vi "calcRigidBodyAuth.vi"(8 "error in (no error)":errorcluster, 10 "Rigid Body Stroke File":string="rbStroke.txt", 11 "OptCtrl in":refnum<class "OptCtrl.lvclass">) -> (0 "error out":errorcluster, 2 "Authority (1 um)":dbl[](array[numeric]), 3 "OptCtrl out":refnum<class "OptCtrl.lvclass">)   [LabVIEW 2016, in "OfcFunc.lvlib" / "OptCtrl.lvclass"]
doc: "Calculate the distribution of control authority of rigid body."
uses:
  OptCtrl.lvclass
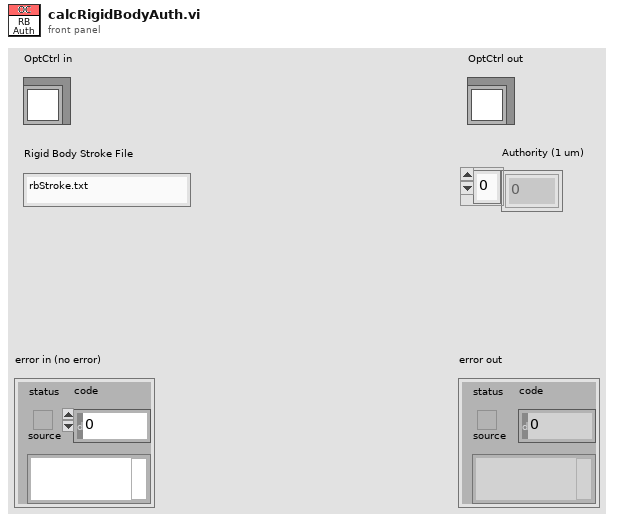
[diagram p1: front panel]
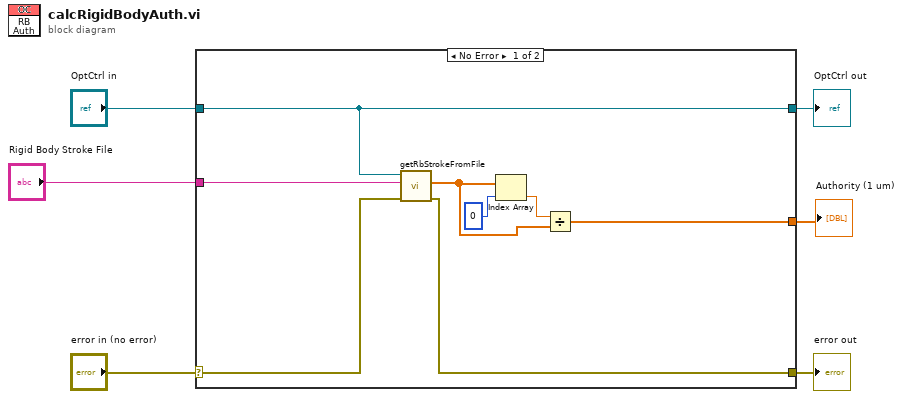
[diagram p0: block diagram]
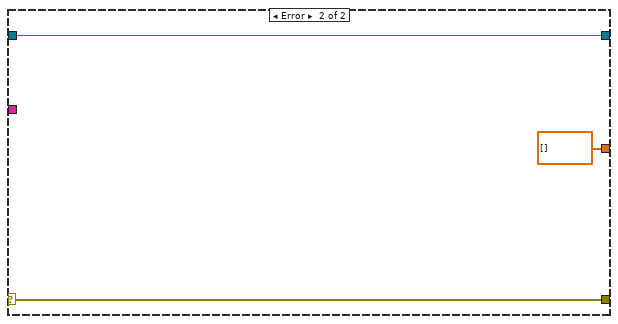
[diagram p2: hidden frame]
diagram:
  n1 = case shown="No Error" "error in (no error)" {
    selector: "error in (no error)" -> [w8 w17]
    tunnel: [w7 w17] -> w5
    tunnel: [w11 w16] -> w3
    tunnel: "OptCtrl in" -> [w11 w16]
    tunnel: "Rigid Body Stroke File" -> [w10 _]
    tunnel: [w12 dbl[] []] -> w1
    frame No Error {
      n2 = call "getRbStrokeFromFile.vi"("error in (no error)"=w8, "Rigid Body Stroke File"=w10, "OptCtrl in"=w11) -> ("error out"=w7:errorcluster, "Stroke in Um"=w9:dbl[])  [unwired: 6 in, 1 out]
      n3 = Index Array(array=w9, index=0) -> (element=w13:dbl)
      n4 = Divide(x=w13, y=w9) -> (x/y=w12:dbl[])
    }
    frame Error {
    }
  }
  "error out" <- w5
  "OptCtrl out" <- w3
  "Authority (1 um)" <- w1
